vi "Cargar Refrescos y Papas.vi"(7 "REFRESCOS Y PAPAS ACTOR in":refnum<class "REFRESCOS Y PAPAS ACTOR.lvclass">, 11 "MulticolumnListbox in":refnum<vi>) -> ()   [LabVIEW 2019, in "REFRESCOS Y PAPAS ACTOR.lvlib" / "REFRESCOS Y PAPAS ACTOR.lvclass"]
uses:
  REFRESCOS Y PAPAS ACTOR.lvclass
  REFRESCOS Y PAPAS ACTOR.lvclass/REFRESCOS Y PAPAS ACTOR.ctl
  <vilib>/Utility/config.llb/Read Key (Double).vi
  <vilib>/Utility/config.llb/Read Key (String).vi
  <vilib>/Utility/config.llb/NI_LVConfig.lvlib
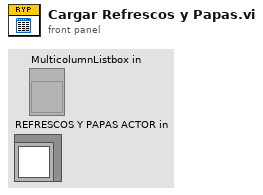
[diagram p1: front panel]
types:
  T1 = typedef "NI_LVConfig.lvlib/Config Data RefNum.ctl" = refnum<k1>
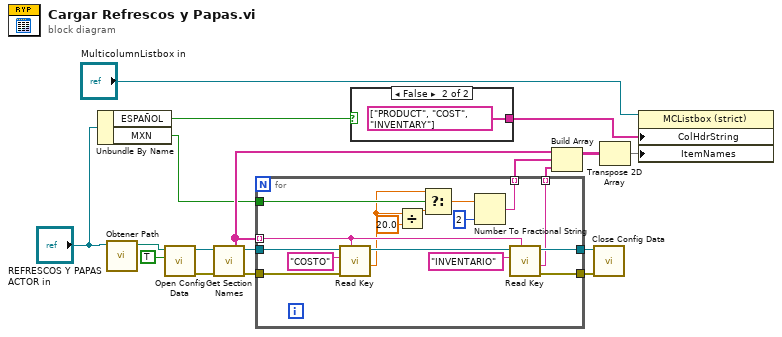
[diagram p0: block diagram]
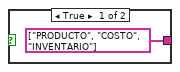
[diagram p2: hidden frame]
diagram:
  n1 = Unbundle By Name("REFRESCOS Y PAPAS ACTOR in") -> ("ESPAÑOL"=w4:bool, "MXN"=w2:bool)
  n2 = call "Obtener Path.vi"("REFRESCOS Y PAPAS ACTOR in"="REFRESCOS Y PAPAS ACTOR in") -> ("appended path"=w18:path)  [unwired: 10 in]
  n3 = call <vilib>:"Open Config Data.vi"("create file if necessary (T)"=TRUE, "configuration file path"=w18) -> ("error out"=w16:errorcluster, "refnum"=w15:T1)  [unwired: 7 in, 1 out]
  n4 = call <vilib>:"Get Section Names.vi"("error in (no error)"=w16, "refnum"=w15) -> ("error out"=w13:errorcluster, "section names"=w8:string[], "refnum out"=w14:T1)  [unwired: 7 in]
  n5 = for {
    tunnel: w14 -> [w34]
    tunnel: w13 -> [w33]
    tunnel: w8 -> [w26] mode=indexing
    tunnel: [w29] -> w12
    tunnel: [w28] -> w11
    tunnel: [w27] -> w9 mode=indexing
    tunnel: w2 -> [w21]
    tunnel: [w19] -> w1 mode=indexing
    n6 = call-poly <vilib>:"Read Key.vi"("section"=w26, "error in (no error)"=w33, "key"="COSTO", "refnum"=w34) -> ("value"=w20:dbl, "refnum out"=w31:T1)  [unwired: 4 in, 2 out]
    n7 = Divide(x=w20, y=20.0) -> (x/y=w25:dbl)
    n8 = Select(t=w20, s=w21, f=w25) -> (s? t:f=w23:dbl)
    n9 = Number To Fractional String(number=w23, precision (6)=i16 2) -> (F-format string=w19:string)  [unwired: 2 in]
    n10 = call-poly <vilib>:"Read Key.vi"("section"=w26, "key"="INVENTARIO", "refnum"=w31) -> ("error out"=w29:errorcluster, "value"=w27:string, "refnum out"=w28:T1)  [unwired: 5 in, 1 out]
  }
  n11 = case shown="False" w4 {
    tunnel: [string[] ["PRODUCTO", "COSTO", "INVENTARIO"] ("Column Header Strings[]") string[] ["PRODUCT", "COST", "INVENTARY"] ("Column Header Strings[]")] -> w10
    frame True {
    }
    frame False {
    }
  }
  n12 = Build Array(w8, w1, w9) -> (w7:string[][])
  n13 = call <vilib>:"Close Config Data.vi"("error in (no error)"=w12, "refnum"=w11) -> ()  [unwired: 8 in, 2 out]
  n14 = Transpose 2D Array(2D array=w7) -> (transposed array=w6:string[][])
  n15 = property class="MCListbox (strict)"(reference="MulticolumnListbox in", "ColHdrString"=w10, "ItemNames"=w6) -> ()  [unwired: 1 in, 2 out]
